vi "meaSureit_SPCM.vi"() -> ()   [LabVIEW 2013]
uses:
  <vilib>/DAQmx/read.llb/DAQmx Read (Analog DBL 1Chan 1Samp).vi
  <vilib>/DAQmx/write.llb/DAQmx Write (Analog DBL 1Chan 1Samp).vi
  <vilib>/DAQmx/read.llb/DAQmx Read (Analog 1D DBL NChan 1Samp).vi
  <vilib>/DAQmx/miscellaneous.llb/DAQmx Fill In Error Info.vi
  <vilib>/Utility/file.llb/Write To Spreadsheet File (DBL).vi
  Instance           2 17Saved   meaSureit .vi
panel:
  in  "Switched":bool=TRUE
  out "Elapsed Time (s)":dbl=22.996299266815186
  in  "Wait time":dbl=60.0 caption="Time Target (s)"
  in  "Auto measurement?":bool
  in  "# sweeps to do":dbl=5.0
  out "Sweeps Completed":dbl
  in  "Sweep":bool
  in  "Auto-pick Sens?":bool
  in  "Auto-pick min. sensitivity":T1(ring)=enum."10nA/V"
  in  "Multiscan Ramp time":dbl=0.5
  in  "Sens Change wait time (ms)":u32=500
  in  "Detect Sens?":bool=TRUE
  in  "Preamp Bias (mv)":i32=-25
  in  "Preamp Bias on?":bool
  in  "Preamp resource":refnum<visa-resource-name>="COM14"
  in  "Preamp Sensitivity":T1(ring)=enum."10nA/V"
  in  "Direction":bool=TRUE
  in  "Cont. Update":bool=TRUE
  out "Error":errorcluster
  in  "Print":bool
  in  "Pause":bool=TRUE caption="Run"
  out "Extension":i32 format="%03.0f"
  in  "Path":path=path "C:/Users/aspitarl/Desktop/a"
  in  "Autosave":bool caption="+"
  in  "Tab Control":T2(tab)
  in  "Parameters":T3={"min"=-10.0, "max"=10.0, "step"=0.03, "speed (steps/s)"=100.0, "Stop at \nthe end"=FALSE} {"step" format="%.5p"; "speed (steps/s)" format="%.2f"; "max" format="%.5p"; "min" format="%.5p"}
  out "end":bool
  in  "Scan Channel 2":u16(ring)=1 items=["Vsd", "Vg", "Time"]
  in  "Scan Channel 3":u16(ring)=1 items=["Vsd", "Vg", "Time"]
  in  "Scan 3":bool caption="+"
  out "value 2":dbl=0.27999999999999997 format="%.5p"
  out "value 3":dbl format="%#.5p"
  in  "delay 3":dbl format="%#.2p"
  in  "delay 2":dbl format="%#.2p"
  in  "Scan":dbl[][](array[numeric])
  out "Value":dbl=0.01000000000002041 format="%#.5p"
  out "graph data":dbl[][](array[numeric]) format="%.2f"
  in  "SaveCFG":bool
  in  "LoadCFG":bool
  in  "update graph":bool=TRUE
  in  "graph bin":dbl=1.0
  out "date":string="Mon, 25 Jul 2016; 13:06"
  out "Data Size":dbl(slide)=228.0 scale=0.0..50000.0 scale format="%.0p"
  in  "Clear":bool
  in  "File Name":string="test"
  in  "Scan Channel":u16(ring)=1 items=["Vsd", "Vg", "Time"]
  in  "Update":bool
  in  "Channels Out":T4(array[cluster])=[{"Channel"=1, "Value"=0.0, "Factor"=1.0, "Name"="Vsd", "min"=-1.0, "max"=1.0, "step"=0.01, "speed"=5.0, "Direction"=TRUE, "Stop at \nthe end"=TRUE}, {"Channel"=2, "Value"=0.01000000000002041, "Factor"=1.0, "Name"="Vg", "min"=-10.0, "max"=10.0, "step"=0.03, "speed"=100.0, "Direction"=TRUE, "Stop at \nthe end"=FALSE}, {"Channel"=0, "Value"=0.0, "Factor"=1.0, "Name"="Time", "min"=0.0, "max"=100000.0, "step"=0.01, "speed"=100.0, "Direction"=FALSE, "Stop at \nthe end"=TRUE}] {"step" format="%.5p"; "speed" format="%.2f"; "max" format="%.5p"; "min" format="%.5p"; "Factor" format="%.2p"; "Value" format="%.5p"}
  out "data":dbl[][](array[numeric]) format="%.2f"
  in  "Y channel":i32(ring) items=["I", "AI2"]
  in  "Save":bool
  out "XY Graph":cluster{dbl[], dbl[]}(graph)
  in  "Quit":bool
  in  "Scan DAQ":bool
  in  "Channels In":T5(array[cluster])=[{"Ring"=1, "Value"=1.691596709266448e-13, "Factor"=1e-09, "Name"="I"}, {"Ring"=2, "Value"=-0.0001533531911967702, "Factor"=1.0, "Name"="AI2"}] {"Factor" format="%.2p"; "Value" format="%.5p"}
  # "speed (steps/sec)"
  # "Direction"
  # "Factor"
  # "Name"
  # "Value"
  # "Factor"
  # "Name"
  # "min"
  # "max"
  # "step"
  # "Value"
  # "Define parameters in the Channels Out Panel"
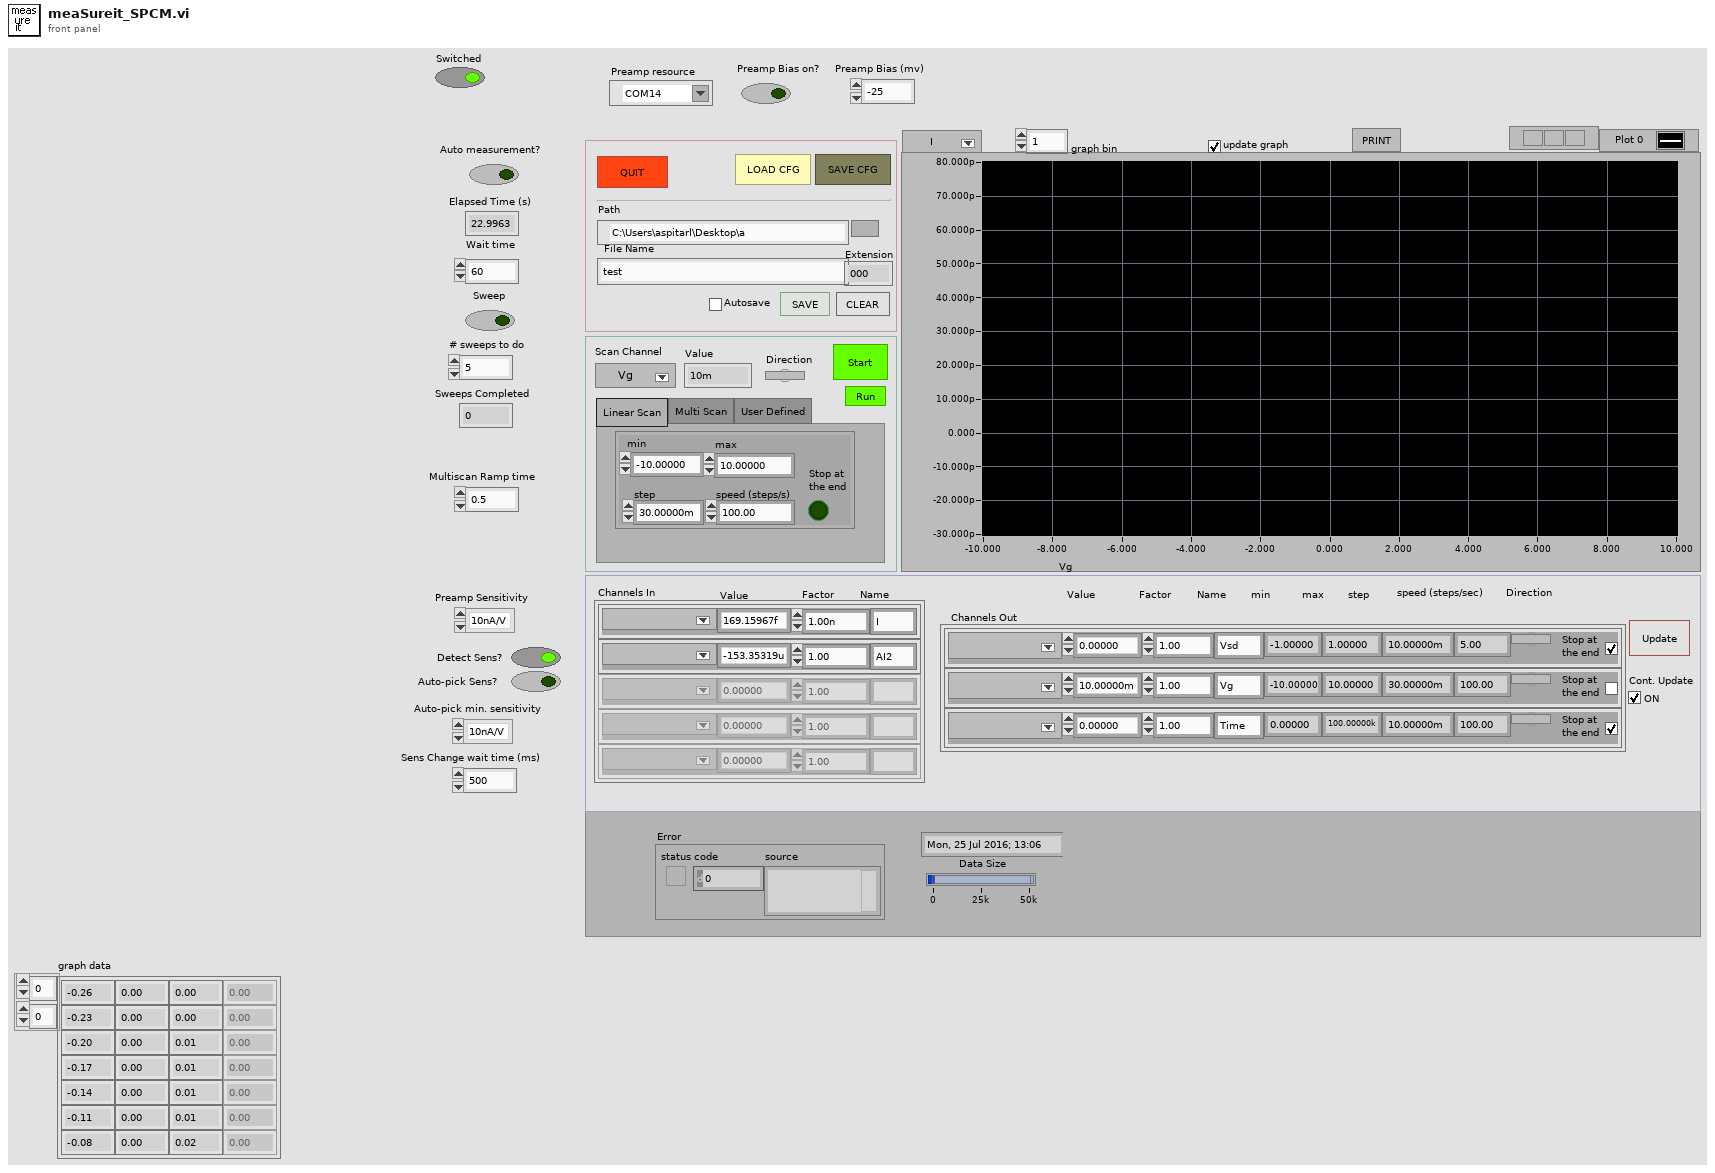
[diagram p1: front panel]
types:
  T1 = enum16{"1pA/V", "2pA/V", "5pA/V", "10pA/V", "20pA/V", "50pA/V", "100pA/V", "200pA/V", "500pA/V", "1nA/V", "2nA/V", "5nA/V", "10nA/V", "20nA/V", "50nA/V", "100nA/V", "200nA/V", "500nA/V", "1uA/V", "2uA/V", "5uA/V", "10uA/V", "20uA/V", "50uA/V", "100uA/V", "200uA/V", "500uA/V", "1mA/V"}
  T2 = enum32{"Linear Scan", "Multi Scan", "User Defined"}
  T3 = cluster{"min":dbl, "max":dbl, "step":dbl, "speed (steps/s)":dbl, "Stop at \nthe end":bool}
  T4 = cluster{"Channel":u16, "Value":dbl, "Factor":dbl, "Name":string, "min":dbl, "max":dbl, "step":dbl, "speed":dbl, "Direction":bool, "Stop at \nthe end":bool}[]
  T5 = cluster{"Ring":u16, "Value":dbl, "Factor":dbl, "Name":string}[]
  T6 = cluster{"Channel":u16, "Value":dbl, "Factor":dbl, "Name":string, "min":dbl, "max":dbl, "step":dbl, "speed":dbl, "direction":bool, "Boolean":bool}[]
  T7 = cluster{"Channel":u16, "Value":dbl, "Factor":dbl, "Name":string}[]
  T8 = cluster{"Channel":u16, "Value":dbl, "Factor":dbl, "Name":string, "min":dbl, "max":dbl, "step":dbl, "speed":dbl, "Direction":bool, "Stop at \nthe end":bool}
  T9 = cluster{"min":dbl, "max":dbl, "step":dbl, "speed (steps/s)":dbl, bool}
  T10 = cluster{void, void, void, void, void, "y":dbl, void, void, void, bool}
  T11 = cluster{void, void, void, void, "y":dbl, void, void, void, void, bool}
  T12 = cluster{void, void, void, void, "y":dbl, void, void, void, void, bool}[]
  T13 = cluster{"Preamp Bias on?":bool, "Preamp Bias (mv)":i32, "Preamp Sensitivity":enum16{"1pA/V", "2pA/V", "5pA/V", "10pA/V", "20pA/V", "50pA/V", "100pA/V", "200pA/V", "500pA/V", "1nA/V", "2nA/V", "5nA/V", "10nA/V", "20nA/V", "50nA/V", "100nA/V", "200nA/V", "500nA/V", "1uA/V", "2uA/V", "5uA/V", "10uA/V", "20uA/V", "50uA/V", "100uA/V", "200uA/V", "500uA/V", "1mA/V"}, "Detect Sens?":bool, "Sens Change wait time (ms)":u32, "Auto-pick min. sensitivity":enum16{"1pA/V", "2pA/V", "5pA/V", "10pA/V", "20pA/V", "50pA/V", "100pA/V", "200pA/V", "500pA/V", "1nA/V", "2nA/V", "5nA/V", "10nA/V", "20nA/V", "50nA/V", "100nA/V", "200nA/V", "500nA/V", "1uA/V", "2uA/V", "5uA/V", "10uA/V", "20uA/V", "50uA/V", "100uA/V", "200uA/V", "500uA/V", "1mA/V"}, "Auto-pick Sens?":bool}
  T14 = cluster{"min":dbl, "max":dbl, "step":dbl, "speed":dbl, "Stop at \nthe end":bool}
  T15 = cluster{"y":dbl, "max":dbl, "step":dbl, "speed (steps/s)":dbl, bool}
  T16 = cluster{"min":dbl, "y":dbl, "step":dbl, "speed (steps/s)":dbl, bool}
  T17 = cluster{"Ring":u16, "Value":dbl, "Factor":dbl, "Name":string}
  T18 = cluster{"Channel":u16, "Value":dbl, "Factor":dbl, "Name":string, "min":dbl, "max":dbl, "step":dbl, "speed":dbl, "Direction":bool, "Stop at the end":bool}[]
  T19 = cluster{"Channel":u16, "Value":dbl, "Factor":dbl, "Name":string, "min":dbl, "max":dbl, "step":dbl, "speed":dbl, "Direction":bool, "Stop at the end":bool}
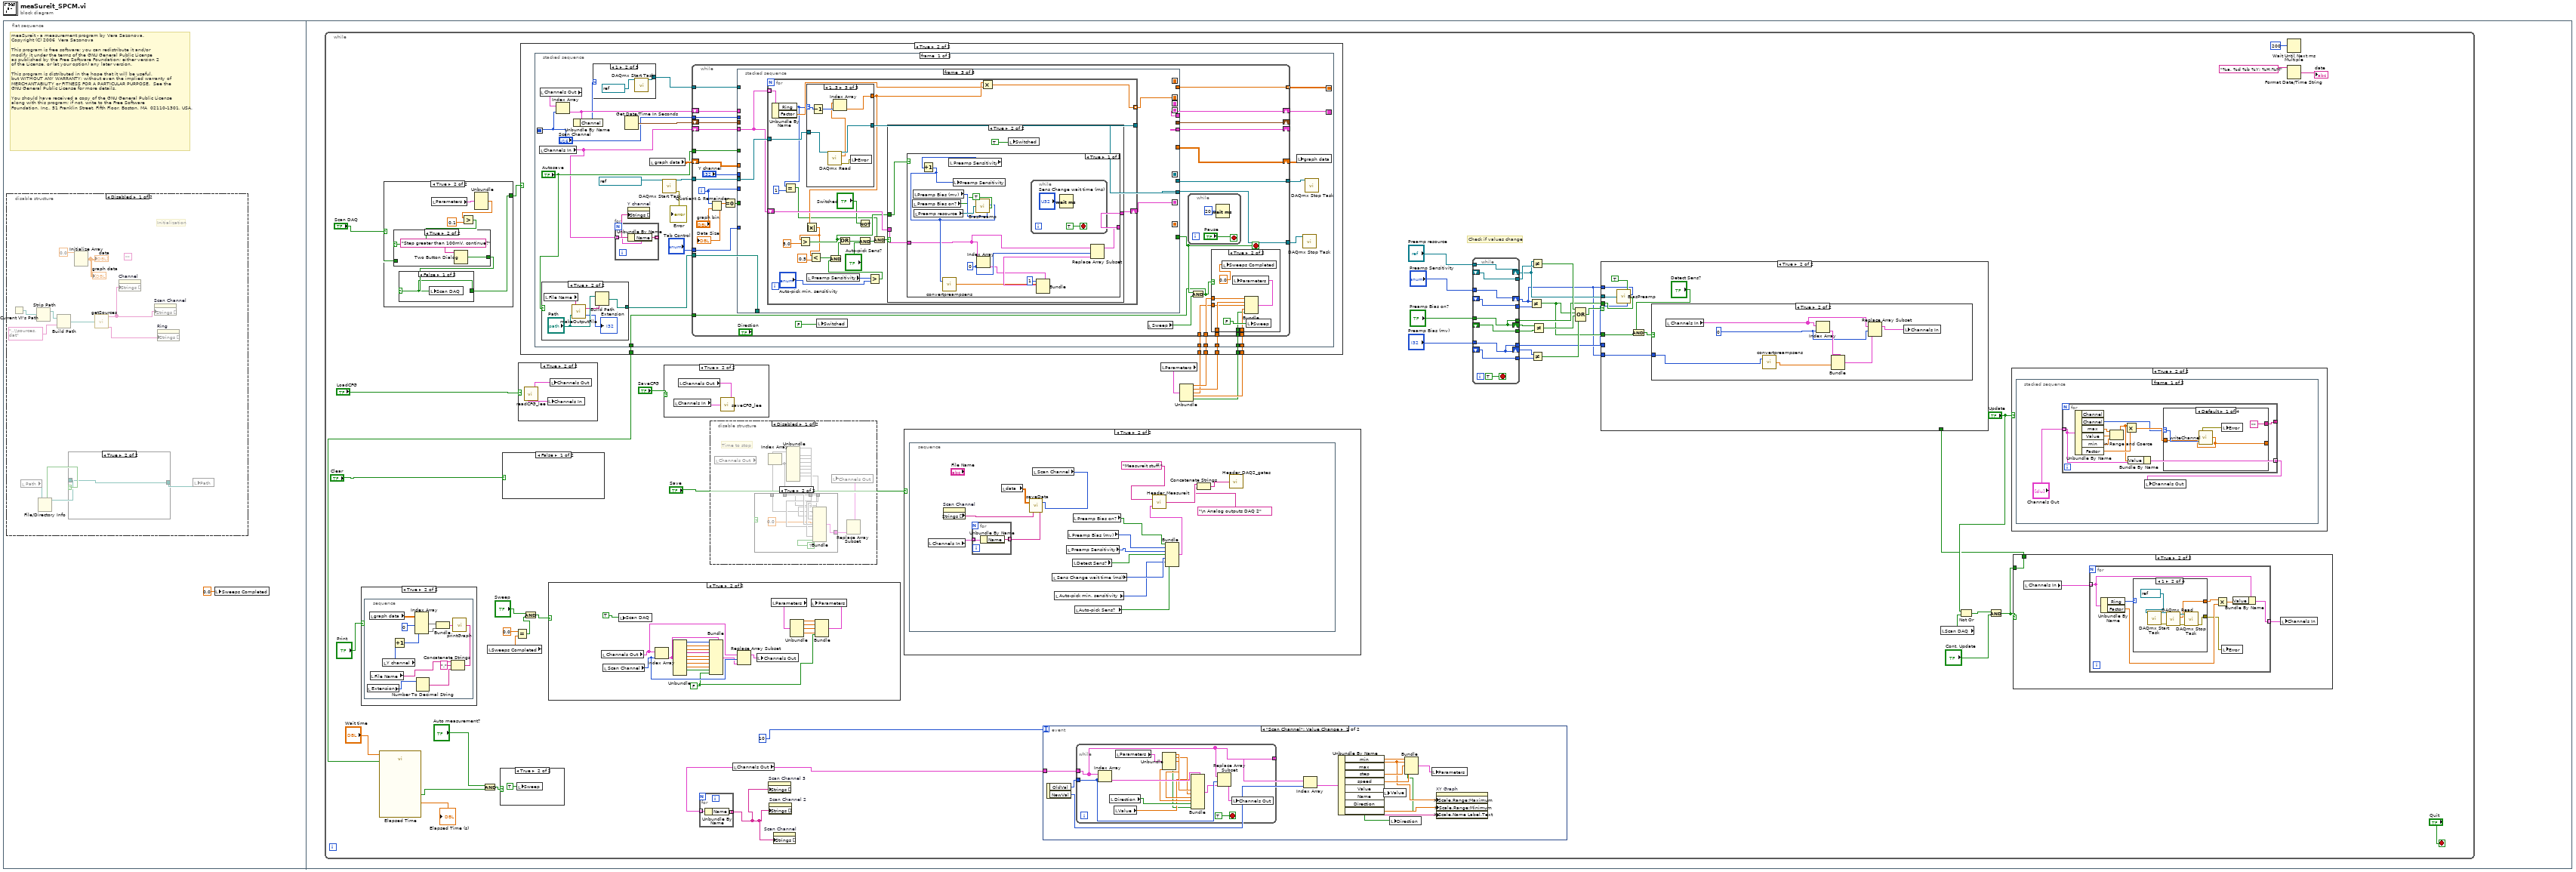
[diagram p0: block diagram]
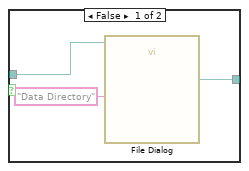
[diagram p2: hidden frame]
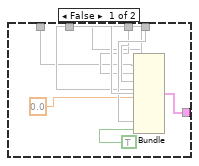
[diagram p5: hidden frame]
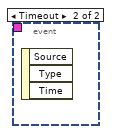
[diagram p13: hidden frame]
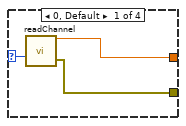
[diagram p15: hidden frame]
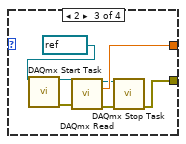
[diagram p16: hidden frame]
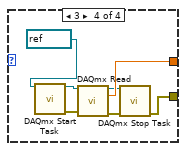
[diagram p17: hidden frame]
diagram:
  n1 = flat-sequence {
    frame #0 {
      # "meaSureit - a measurement program by Vera Sazonova.\nCopyright (C) 2006  Vera Sazonova\n\nThis program is free software; you can redistribute it and/or\nmodify it under the terms of the GNU General Public License\nas published by the Free Software Foundation; either version 2\nof the License, or (at your option) any later version.\n\nThis program is distributed in the hope that it will be useful,\nbut WITHOUT ANY WARRANTY; without even the implied warranty of\nMERCHANTABILITY or FITNESS FOR A PARTICULAR PURPOSE.  See the\nGNU General Public License for more details.\n\nYou should have received a copy of the GNU General Public License\nalong with this program; if not, write to the Free Software\nFoundation, Inc., 51 Franklin Street, Fifth Floor, Boston, MA  02110-1301, USA."
      n2 = disable-structure shown="Disabled" {
        frame Disabled {
          (unwired) ""
          # "Initialization"
          n3 = Current VI's Path() -> (path=w11:path)
          n4 = local read "Path"() -> (w6:path)
          n5 = Strip Path(path=w11) -> (stripped path=w10:path)  [unwired: 1 out]
          n6 = File/Directory Info(path=w6) -> (path out=w4:path, directory=w5:bool)  [unwired: 1 in, 5 out]
          n7 = Build Path(base path=w10, name or relative path="..\\sources.dat") -> (appended path=w2:path)
          n8 = case shown="True" w5 {
            tunnel: w4 -> [w16 w17]
            tunnel: [w15 w17] -> w3
            frame False {
              n9 = call "File Dialog"("start path"=w16, "prompt"="Data Directory") -> ("selected path"=w15:path)  [unwired: 5 in, 8 out]
            }
            frame True {
            }
          }
          n10 = Initialize Array(0.0) -> (→"data" →"graph data":dbl[][])  [unwired: 2 out]
          n11 = call "getSources.vi"("Path"=w2) -> ("Output Sources"=w7:string[], "Input Sources"=w8:string[])  [unwired: 2 out]
          n12 = property on="Channel" class="Ring (strict)"("Strings []"=w7) -> ()  [unwired: 2 in, 2 out]
          n13 = property on="Scan Channel" class="Ring (strict)"("Strings []"=w7) -> ()  [unwired: 2 in, 2 out]
          n14 = property on="Ring" class="Ring (strict)"("Strings []"=w8) -> ()  [unwired: 2 in, 2 out]
          n15 = local write "Path"(w3) -> ()
        }
        frame Enabled {
        }
      }
      n16 = local write "Sweeps Completed"(0.0 ("Number of sweeps")) -> ()
    }
    frame #1 {
      n17 = while {
        stop <- "Quit" stop-if-true
        # "Check if values change"
        n18 = case shown="True" "Print" {
          frame False {
          }
          frame True {
            n19 = stacked-sequence {
              frame #0 {
                n20 = local read "Extension"() -> (w243:i32)
                n21 = local read "graph data"() -> (w246:dbl[][])
                n22 = local read "File Name"() -> (w242:string)
                n23 = local read "Y channel"() -> (w245:i32)
                n24 = Increment(x=w245) -> (x+1=w247:i32)
                n25 = Index Array(array=w246, index (col) #1=0, index (col) #2=w247) -> (element #1=w250:dbl[], element #2=w249:dbl[])  [unwired: 2 in]
                n26 = Number To Decimal String(number=w243) -> (decimal integer string=w240:string)  [unwired: 1 out]
                n27 = Bundle("graph data"=w250, "graph data"=w249) -> (w244:cluster{"graph data":dbl[], "graph data":dbl[]})  [unwired: 1 out]
                n28 = Concatenate Strings(w242, "." ("string"), w240) -> (w239:string)
                n29 = call "printGraph.vi"("File"=w239, "XY Graph 2"=w244) -> ()
              }
            }
          }
        }
        n30 = case shown="True" "Scan DAQ" {
          selector: "Scan DAQ" -> [w136 w139]
          tunnel: [w136 w137] -> w35
          frame False {
          }
          frame True {
            n31 = local read "Parameters"() -> (w143:T3)
            n32 = Unbundle(w143) -> ("step"=w142:dbl)  [unwired: 4 out]
            n33 = Greater?(x=w142, y=0.1) -> (0:w140:bool)
            n34 = case shown="True" w140 {
              tunnel: [w146 w147] -> w138
              tunnel: w139 -> [w146 _]
              frame False {
              }
              frame True {
                n35 = Two Button Dialog(message="Step greater than 100mV, continue?") -> (T button?=w147:bool)  [unwired: 2 in]
              }
            }
            n36 = case shown="False" w138 {
              selector: w138 -> [w144 w145]
              tunnel: [w144 w145] -> w137
              frame False {
                n37 = local write "Scan DAQ"(w144) -> ()
              }
              frame True {
              }
            }
          }
        }
        n38 = local read "Sweeps Completed"() -> (w33:dbl)
        n39 = case shown="False" "Clear" {
          frame False {
          }
          frame True {
            w256 = 0.0
            n40 = local write "Data Size"(w256) -> ()
            n41 = Initialize Array(w256) -> (w255:dbl[][])  [unwired: 2 out]
            n42 = local write "graph data"(w255) -> ()
            n43 = local write "data"(w255) -> ()
          }
        }
        n44 = Equal?(x=0.0, y=w33) -> (x = y?=w31:bool)
        n45 = case shown="True" "LoadCFG" {
          frame False {
          }
          frame True {
            n46 = call "readCFG_lee.vi"() -> ("Channels Out"=w254:T6, "Channels In"=w253:T7)  [unwired: 1 in]
            n47 = local write "Channels In"(w253) -> ()
            n48 = local write "Channels Out"(w254) -> ()
          }
        }
        n49 = And(x="Sweep", y=w31) -> (x .and. y?=w34:bool)
        n50 = case shown="True" w34 {
          frame False {
          }
          frame True {
            w115 = FALSE
            n51 = local read "Channels Out"() -> (w123:T4)
            n52 = local read "Scan Channel"() -> (w125:u16)
            n53 = local write "Scan DAQ"(TRUE) -> ()
            n54 = Index Array(array=w123, index=w125) -> (element=w116:T8)
            n55 = Unbundle(w116) -> ("Channel"=w126:u16, "Value"=w127:dbl, "Factor"=w128:dbl, "Name"=w129:string, "min"=w130:dbl, "max"=w131:dbl, "step"=w132:dbl, "speed"=w133:dbl, "Direction"=w134:bool)  [unwired: 1 out]
            n56 = Bundle(cluster=w116, "Channel"=w126, "Value"=w127, "Factor"=w128, "Name"=w129, "min"=w130, "max"=w131, "step"=w132, "speed"=w133, "Direction"=w134, "Stop at \nthe end"=w115) -> (w124:T8)
            n57 = Replace Array Subset(array=w123, new element=w124, index=w125) -> (w122:T4)
            n58 = local write "Channels Out"(w122) -> ()
            n59 = local read "Parameters"() -> (w121:T3)
            n60 = Unbundle(w121) -> ("min"=w118:dbl, "max"=w119:dbl, "step"=w120:dbl, "speed (steps/s)"=w117:dbl)  [unwired: 1 out]
            n61 = Bundle("min"=w118, "max"=w119, "step"=w120, "speed (steps/s)"=w117, w115) -> (w114:T9)  [unwired: 1 in]
            n62 = local write "Parameters"(w114) -> ()
          }
        }
        n63 = case shown="True" "SaveCFG" {
          frame False {
          }
          frame True {
            n64 = local read "Channels In"() -> (w251:T5)
            n65 = local read "Channels Out"() -> (w252:T4)
            n66 = call "saveCFG_lee.vi"("Channels Out"=w252, "Channels In"=w251) -> ()
          }
        }
        n67 = disable-structure shown="Disabled" {
          frame Disabled {
            # "Time to stop"
            n68 = local read "Channels Out"() -> (w88:T4)
            n69 = Index Array() -> (element=w75)  [unwired: 2 in]
            n70 = Unbundle(w75) -> (w83, w84, w82, w81, w80, w79, w78, w77, w76)  [unwired: 1 out]
            n71 = case shown="True" {
              selector: _ -> [_ _]
              tunnel: w75 -> [w101 w113]
              tunnel: w76 -> [w100 w112]
              tunnel: w77 -> [w99 w111]
              tunnel: w78 -> [w98 w110]
              tunnel: w79 -> [_ w109]
              tunnel: w80 -> [w97 _]
              tunnel: w81 -> [w96 w108]
              tunnel: w82 -> [w95 w107]
              tunnel: w83 -> [w94 w106]
              tunnel: w84 -> [w92 w104]
              tunnel: [w90 w102] -> w85
              frame False {
                n72 = Bundle(cluster=w101, w94, w92, w95, w96, w97, "y"=0.0, w98, w99, w100, TRUE) -> (w90:T10)
              }
              frame True {
                n73 = Bundle(cluster=w113, w106, w104, w107, w108, "y"=0.0, w109, w110, w111, w112, TRUE) -> (w102:T11)
              }
            }
            n74 = Replace Array Subset(new element=w85) -> (array=w87:T12, w89:T12, index=w86:i32)
            n75 = local write "Channels Out"(w89) -> ()
          }
          frame Enabled {
          }
        }
        n76 = local read "Channels Out"() -> (w59:T4)
        n77 = for {
          tunnel: w59 -> [w203] mode=indexing
          tunnel: [w202] -> w58 mode=indexing
          n78 = Unbundle By Name(w203) -> ("Name"=w202:string)
        }
        n79 = property on="Scan Channel 3" class="Ring (strict)"("Strings []"=w58) -> ()  [unwired: 2 in, 2 out]
        n80 = property on="Scan Channel 2" class="Ring (strict)"("Strings []"=w58) -> ()  [unwired: 2 in, 2 out]
        n81 = property on="Scan Channel" class="Ring (strict)"("Strings []"=w58) -> ()  [unwired: 2 in, 2 out]
        n82 = case shown="True" "Save" {
          frame False {
          }
          frame True {
            n83 = stacked-sequence {
              frame #0 {
                n84 = local read "Channels In"() -> (w328:T5)
                n85 = property on="Scan Channel" class="Ring (strict)"() -> ("Strings []"=w330:string[])  [unwired: 2 in, 2 out]
                n86 = for {
                  tunnel: w328 -> [w332] mode=indexing
                  tunnel: [w331] -> w327 mode=indexing
                  n87 = Unbundle By Name(w332) -> ("Name"=w331:string)
                }
                n88 = local read "data"() -> (w329:dbl[][])
                n89 = local read "Scan Channel"() -> (w326:u16)
                n90 = call "saveData.vi"("Names  In"=w327, "Channel"=w326, "Names  Out"=w330, "Data"=w329) -> ()
                n91 = local read "Sens Change wait time (ms)"() -> (w319:u32)
                n92 = local read "Auto-pick min. sensitivity"() -> (w318:T1)
                n93 = local read "Preamp Sensitivity"() -> (w322:T1)
                n94 = local read "Preamp Bias (mv)"() -> (w323:i32)
                n95 = local read "Detect Sens?"() -> (w321:bool)
                n96 = local read "Preamp Bias on?"() -> (w324:bool)
                n97 = local read "Auto-pick Sens?"() -> (w317:bool)
                n98 = Bundle("Preamp Bias on?"=w324, "Preamp Bias (mv)"=w323, "Preamp Sensitivity"=w322, "Detect Sens?"=w321, "Sens Change wait time (ms)"=w319, "Auto-pick min. sensitivity"=w318, "Auto-pick Sens?"=w317) -> (w320:T13)  [unwired: 1 in]
                n99 = call "Header_Measureit.vi"("Cluster"=w320, "String in"="Measureit stuff:") -> ("String out"=w316:string)
                n100 = Concatenate Strings(w316, "\n Analog outputs DAQ 2") -> (w314:string)
                n101 = call "Header_DAQ2_gates.vi"("String in"=w314) -> ()  [unwired: 1 out]
              }
            }
          }
        }
        n102 = event shown="[0] \"Scan Channel\": Value Change" {
          selector: _ -> [_ _]
          dyn-events: _ -> [_ _]
          timeout: 10 -> [_ _]
          tunnel: w59 -> [w178 _]
          event "Scan Channel": Value Change {
            n103 = event-data() -> ("OldVal"=w176:u16, "NewVal"=w177:u16)  [unwired: 1 out]
            n104 = while {
              tunnel: w178 -> [w190]
              tunnel: w176 -> [w192]
              tunnel: [w190] -> w175
              stop <- TRUE stop-if-true
              n105 = Index Array(array=w190, index=w192) -> (element=w200:T8)
              n106 = local read "Direction"() -> (w194:bool)
              n107 = local read "Value"() -> (w193:dbl)
              n108 = local read "Parameters"() -> (w199:T3)
              n109 = Unbundle(w199) -> ("min"=w198:dbl, "max"=w197:dbl, "step"=w196:dbl, "speed (steps/s)"=w195:dbl, "Stop at \nthe end"=w188:bool)
              n110 = Bundle(cluster=w200, "Value"=w193, "min"=w198, "max"=w197, "step"=w196, "speed"=w195, "Direction"=w194, "Stop at \nthe end"=w188) -> (w191:T8)  [unwired: 3 in]
              n111 = Replace Array Subset(array=w190, new element=w191, index=w192) -> (w189:T4)
              n112 = local write "Channels Out"(w189) -> ()
            }
            n113 = Index Array(array=w175, index=w177) -> (element=w187:T8)
            n114 = Unbundle By Name(w187) -> ("min"=w181:dbl, "max"=w182:dbl, "step"=w185:dbl, "speed"=w184:dbl, "Value"=w186:dbl, "Name"=w180:string, "Direction"=w179:bool, "Stop at \nthe end"=w174:bool)
            n115 = local write "Value"(w186) -> ()
            n116 = local write "Direction"(w179) -> ()
            n117 = Bundle("min"=w181, "max"=w182, "step"=w185, "speed"=w184, "Stop at \nthe end"=w174) -> (w183:T14)  [unwired: 1 out]
            n118 = local write "Parameters"(w183) -> ()
            n119 = property on="XY Graph" class="XYGraph (strict)"("X Scale.Range:Maximum"=w182, "X Scale.Range:Minimum"=w181, "X Scale.Name Label.Text"=w180) -> ()  [unwired: 2 in, 2 out]
          }
          event Timeout {
            n120 = event-data() -> ()  [unwired: 4 out]
          }
        }
        n121 = local read "Parameters"() -> (w30:T3)
        n122 = Unbundle(w30) -> ("min"=w29:dbl, "max"=w28:dbl, "step"=w27:dbl, "speed (steps/s)"=w26:dbl, "Stop at \nthe end"=w25:bool)
        n123 = case shown="True" w35 {
          tunnel: w29 -> [_ w339]
          tunnel: w28 -> [_ w338]
          tunnel: w27 -> [_ w337]
          tunnel: w26 -> [_ w336]
          tunnel: w25 -> [_ w335]
          tunnel: [FALSE w334] -> w18
          frame False {
          }
          frame True {
            n124 = stacked-sequence {
              seq-local: [w362 _] -> [_ w759]
              seq-local: [w365 _] -> [_ w756]
              seq-local: ["Scan Channel" _] -> [_ w755]
              tunnel: w339 -> [w345 _]
              tunnel: w338 -> [w344 _]
              tunnel: w337 -> [w343 _]
              tunnel: w336 -> [w342 _]
              tunnel: w335 -> [w341 _]
              tunnel: [w340 _] -> w334
              frame #0 {
                n125 = local read "Channels In"() -> (w348:T5)
                n126 = local read "Channels Out"() -> (w353:T4)
                n127 = case shown="True" "Autosave" {
                  tunnel: [path "" ("appended path") w373] -> w349
                  frame False {
                  }
                  frame True {
                    n128 = local read "File Name"() -> (w372:string)
                    n129 = call "makeOutputFile.vi"("Path"="Path", "Name"=w372) -> ("Extension"=→"Extension":i32, "File Name"=w370:string)
                    n130 = Build Path(base path="Path", name or relative path=w370) -> (appended path=w373:path)
                  }
                }
                n131 = Index Array(array=w353, index="Scan Channel") -> (element=w359:T8)
                n132 = Unbundle By Name(w359) -> ("Channel"=w358:u16)
                n133 = case shown="1" w358 {
                  tunnel: ["" w375 w377 w379 w381] -> w361
                  frame 0, Default {
                  }
                  frame 1 {
                    n134 = call <vilib>:"DAQmx Start Task.vi"("task/channels in"=refnum<k21> "AO0") -> ("task out"=w375:refnum<k21>)  [unwired: 1 in, 13 out]
                  }
                  frame 2 {
                    n135 = call <vilib>:"DAQmx Start Task.vi"("task/channels in"=refnum<k21> "AO1") -> ("task out"=w377:refnum<k21>)  [unwired: 1 in, 13 out]
                  }
                  frame 12 {
                    n136 = call <vilib>:"DAQmx Start Task.vi"("task/channels in"=refnum<k21> "AO2") -> ("task out"=w379:refnum<k21>)  [unwired: 1 in, 13 out]
                  }
                  frame 13 {
                    n137 = call <vilib>:"DAQmx Start Task.vi"("task/channels in"=refnum<k21> "AO3") -> ("task out"=w381:refnum<k21>)  [unwired: 1 in, 13 out]
                  }
                }
                n138 = for {
                  tunnel: w348 -> [w367] mode=indexing
                  tunnel: [w366] -> w347 mode=indexing
                  n139 = Unbundle By Name(w367) -> ("Name"=w366:string)
                }
                n140 = Get Date/Time In Seconds() -> (seconds since 1Jan1904=w356:timestamp)
                n141 = property on="Y channel" class="Ring (strict)"("Strings []"=w347) -> ()  [unwired: 2 in, 2 out]
                n142 = local read "graph data"() -> (w364:dbl[][])
                n143 = call <vilib>:"DAQmx Start Task.vi"("task/channels in"=refnum<k21> "AI0, AI1, AI2") -> ("task out"=w355:refnum<k21>, "error out"=→"Error":errorcluster)  [unwired: 1 in, 12 out]
                n144 = while {
                  shift-right: [w396] -> w365
                  shift-left: w359 -> [w414]
                  shift-right: [w393] -> w363
                  shift-left: w364 -> [w413]
                  tunnel: [w392] -> w362 mode=indexing
                  tunnel: w355 -> [w412]
                  shift-right: [w410] -> _
                  shift-left: w348 -> [w411]
                  tunnel: w361 -> [w405]
                  tunnel: [w404] -> w360
                  tunnel: [w403] -> w354
                  tunnel: "Tab Control" -> [w402]
                  tunnel: w349 -> [w400]
                  shift-right: [w398] -> _
                  shift-left: w356 -> [w399]
                  tunnel: "Scan Channel" -> [w397]
                  tunnel: "Autosave" -> [w394]
                  tunnel: w345 -> [w389]
                  tunnel: w344 -> [w388]
                  tunnel: w343 -> [w387]
                  tunnel: w342 -> [w386]
                  tunnel: w341 -> [w385]
                  tunnel: [w384] -> w340
                  i -> [w401]
                  stop <- w391 stop-if-true
                  n145 = Quotient & Remainder(x=w401, y="graph bin") -> (x-y*floor(x/y)=w408:dbl, floor(x/y)=→"Data Size":dbl)
                  n146 = Equal To 0?(x=w408) -> (x = 0?=w407:bool)
                  n147 = stacked-sequence {
                    seq-local: [_ _ w521 _ _ _ _ _] -> [_ _ _ w599 w631 _ _ _]
                    seq-local: [w428 _ _ _ _ _ _ _] -> [_ w496 _ w600 w632 _ _ _]
                    seq-local: [_ w502 _ _ _ _ _ _] -> [_ _ _ _ _ w650 _ _]
                    seq-local: [_ _ _ _ _ w649 _ _] -> [_ _ _ _ _ _ w706 _]
                    seq-local: [w432 _ _ _ _ _ _ _] -> [_ w497 _ _ _ _ _ _]
                    seq-local: [w429 _ _ _ _ _ _ _] -> [_ _ _ _ _ w647 _ _]
                    seq-local: [_ _ w519 _ _ _ _ _] -> [_ _ _ w597 _ _ _ _]
                    tunnel: w414 -> [w439 w504 _ _ _ w645 _ w740]
                    tunnel: w413 -> [_ _ _ w605 _ _ _ _]
                    tunnel: w412 -> [_ _ w523 _ _ _ _ _]
                    tunnel: w411 -> [_ _ w520 _ _ _ _ _]
                    tunnel: [_ _ _ w604 _ _ _ _] -> w410
                    tunnel: w407 -> [_ _ _ w603 _ _ _ _]
                    tunnel: w405 -> [w437 _ _ _ _ w653 w708 _]
                    tunnel: [_ _ _ _ _ w646 _ _] -> w404
                    tunnel: [_ _ w522 _ _ _ _ _] -> w403
                    tunnel: w399 -> [w435 _ _ _ _ w651 w707 _]
                    tunnel: w402 -> [w434 w503 _ _ _ w654 w709 _]
                    tunnel: w401 -> [w433 _ _ _ _ _ _ _]
                    tunnel: w400 -> [_ _ _ _ w630 _ _ _]
                    tunnel: [_ _ _ _ _ _ _ w744] -> w391
                    tunnel: [_ _ _ _ _ w652 _ _] -> w398
                    tunnel: w397 -> [_ _ _ _ w629 _ _ _]
                    tunnel: [_ _ _ _ _ _ w705 _] -> w396
                    tunnel: "Y channel" -> [_ _ _ w602 _ _ _ _]
                    tunnel: w394 -> [_ _ _ _ w628 _ _ _]
                    tunnel: [_ _ _ w601 _ _ _ _] -> w393
                    tunnel: [_ _ _ w598 _ _ _ _] -> w392
                    frame #0 {
                      # "stop signal after specified number of sweeps"
                      # "Update Values out Indicator"
                      n148 = Unbundle By Name(w439) -> ("Channel"=w438:u16, "Factor"=w431:dbl)
                      n149 = case shown="\"Linear Scan\", Default" w434 {
                        tunnel: [w469 w473 w475] -> w427
                        tunnel: w439 -> [w466 w472 _]
                        tunnel: [w468 w474 w481] -> w430
                        tunnel: [w467 w471 w480] -> w432
                        tunnel: w433 -> [_ _ w476]
                        frame "Linear Scan", Default {
                          n150 = local read "Direction"() -> (w465:bool)
                          n151 = Unbundle By Name(w466) -> ("speed"=w467:dbl)
                          n152 = Bundle By Name(cluster=w466, "Direction"=w465) -> (w464:T8)
                          n153 = call "update_in_scan_Lee.vi"("Parameters"=w464) -> ("Value"=w468:dbl, "end"=w469:bool, "new direction"=w463:bool)
                          n154 = local write "Direction"(w463) -> ()
                        }
                        frame "Multi Scan" {
                          n155 = Unbundle By Name(w472) -> ("speed"=w471:dbl)
                          n156 = call "update_in_scan_Lee.vi"("Parameters"=w472) -> ("Value"=w474:dbl, "end"=w473:bool, "new direction"=w470:bool)
                          n157 = local write "Direction"(w470) -> ()
                        }
                        frame "User Defined" {
                          n158 = Index Array(array="Scan", index (row) #1=w476, index (col) #1=0 ("disabled index (col)"), index (row) #2=w476, index (col) #2=1 ("disabled index (col)")) -> (element #1=w481:dbl, element #2=w480:dbl)
                          n159 = Array Size(array="Scan") -> (size(s)=w478:i32[])
                          n160 = Index Array(array=w478) -> (element=w477:i32)  [unwired: 1 in]
                          n161 = Greater?(x=w477, y=w476) -> (0:w475:bool)
                        }
                      }
                      "end" <- w427
                      n162 = Multiply(x=w431, y=w430) -> (x*y=w436:dbl)
                      n163 = case shown="1, 2, 12, 13" w438 {
                        selector: w438 -> [w486 _ _]
                        tunnel: w437 -> [_ _ w495]
                        tunnel: ["" "" w494] -> w429
                        tunnel: w436 -> [w485 _ w493]
                        tunnel: [w485 w488 w493] -> w428
                        tunnel: w435 -> [_ w489 _]
                        frame Default {
                          n164 = call "writeChannel.vi"("Value"=w485, "Channel"=w486) -> ("error out"=w484:errorcluster)
                          n165 = local write "Error"(w484) -> ()
                        }
                        frame 0 {
                          n166 = Get Date/Time In Seconds() -> (seconds since 1Jan1904=w490:timestamp)
                          n167 = Subtract(x=w490, y=w489) -> (x-y=w488:dbl)
                        }
                        frame 1, 2, 12, 13 {
                          n168 = call-poly <vilib>:"DAQmx Write.vi"("task/channels in"=w495, "data"=w493) -> ("task out"=w494:refnum<k21>, "error out"=w492:errorcluster)  [unwired: 2 in, 10 out]
                          n169 = local write "Error"(w492) -> ()
                        }
                      }
                      "Value" <- w428
                      n170 = local read "Sweep"() -> (w426:bool)
                      n171 = And(x=w427, y=w426) -> (x .and. y?=w425:bool)
                      n172 = case shown="True" w425 {
                        tunnel: w428 -> [_ w440]
                        frame False {
                        }
                        frame True {
                          n173 = local read "Sweeps Completed"() -> (w445:dbl)
                          n174 = Add(x=w445, y=1.0) -> (x+y=w441:dbl)
                          "Sweeps Completed" <- w441
                          n175 = local write "Sweeps Completed"(w441) -> ()
                          n176 = Greater Or Equal?(x=w441, y="# sweeps to do") -> (x >= y?=w442:bool)
                          n177 = case shown="True" w442 {
                            tunnel: w440 -> [_ w447]
                            frame False {
                            }
                            frame True {
                              n178 = Greater?(x=w447, y=0.0) -> (0:w446:bool)
                              n179 = case shown="True" w446 {
                                frame True {
                                n180 = local read "Parameters"() -> (w455:T3)
                                n181 = Unbundle(w455) -> ("max"=w453:dbl, "step"=w454:dbl, "speed (steps/s)"=w452:dbl)  [unwired: 2 out]
                                n182 = Bundle("y"=0.0, "max"=w453, "step"=w454, "speed (steps/s)"=w452, TRUE) -> (w451:T15)  [unwired: 1 in]
                                n183 = local write "Parameters"(w451) -> ()
                                }
                                frame False {
                                n184 = local read "Parameters"() -> (w462:T3)
                                n185 = Unbundle(w462) -> ("min"=w460:dbl, "step"=w461:dbl, "speed (steps/s)"=w459:dbl)  [unwired: 2 out]
                                n186 = Bundle("min"=w460, "y"=0.0, "step"=w461, "speed (steps/s)"=w459, TRUE) -> (w458:T16)  [unwired: 1 in]
                                n187 = local write "Parameters"(w458) -> ()
                                }
                              }
                            }
                          }
                        }
                      }
                    }
                    frame #1 {
                      n188 = case shown="\"Linear Scan\"" w503 {
                        tunnel: w504 -> [w510 w515 w518]
                        tunnel: [w509 w515 w517] -> w502
                        tunnel: w496 -> [w507 _ w516]
                        frame "Linear Scan" {
                          n189 = local read "Direction"() -> (w506:bool)
                          n190 = Unbundle("Parameters") -> ("min"=w512:dbl, "max"=w513:dbl, "step"=w514:dbl, "speed (steps/s)"=w508:dbl, "Stop at \nthe end"=w505:bool)
                          n191 = Bundle(cluster=w510, "Value"=w507, "min"=w512, "max"=w513, "step"=w514, "speed"=w508, "Direction"=w506, "Stop at \nthe end"=w505) -> (w509:T8)  [unwired: 3 out]
                        }
                        frame "User Defined", Default {
                        }
                        frame "Multi Scan" {
                          n192 = Bundle(cluster=w518, "Value"=w516) -> (w517:T8)  [unwired: 9 out]
                        }
                      }
                      n193 = Divide(x=1000, y=w497) -> (x/y=w501:dbl)
                      n194 = Max & Min(x=w501, y=10.0) -> (max(x,y)=w498:dbl)  [unwired: 1 out]
                      n195 = Wait (ms)(milliseconds to wait=w498) -> ()  [unwired: 1 out]
                    }
                    frame #2 {
                      n196 = for {
                        tunnel: w520 -> [w548] mode=indexing
                        tunnel: w523 -> [w546]
                        tunnel: [w545] -> w522
                        tunnel: [w542] -> w521 mode=indexing
                        shift-right: [w544] -> w519
                        shift-left: w520 -> [w543]
                        n197 = Unbundle By Name(w548) -> ("Ring"=w526:u16, "Factor"=w547:dbl)
                        n198 = Equal?(x=w526, y=u16 1) -> (x = y?=w524:bool)
                        n199 = case shown="1..3" w526 {
                          selector: w526 -> [w587 _ w596]
                          tunnel: [w586 0 w595] -> w532
                          tunnel: w546 -> [w584 w588 w593]
                          tunnel: [w584 w588 w592] -> w545
                          frame Default {
                            n200 = call "readChannel.vi"("Channel"=w587) -> ("Value"=w586:dbl, "error out"=w585:errorcluster)
                            n201 = local write "Error"(w585) -> ()
                          }
                          frame 0 {
                          }
                          frame 1..3 {
                            n202 = Decrement(x=w596) -> (x-1=w594:u16)
                            n203 = call-poly <vilib>:"DAQmx Read.vi"("task/channels in"=w593) -> ("task out"=w592:refnum<k21>, "data"=w591:dbl[], "error out"=w590:errorcluster)  [unwired: 1 in, 11 out]
                            n204 = Index Array(array=w591, index=w594) -> (element=w595:dbl)
                            n205 = local write "Error"(w590) -> ()
                          }
                        }
                        n206 = Absolute Value(x=w532) -> (abs(x)=w531:dbl)
                        n207 = Greater?(x=w531, y=5.0) -> (0:w533:bool)
                        n208 = local read "Preamp Sensitivity"() -> (w535:T1)
                        n209 = Less?(x=w531, y=0.5) -> (x < y?=w537:bool)
                        n210 = Not(x="Switched") -> ()  [unwired: 1 out]
                        n211 = Greater?(x=w535, y="Auto-pick min. sensitivity") -> (0:w538:bool)
                        n212 = And(x=w537, y=w538) -> (x .and. y?=w536:bool)
                        n213 = Or(x=w533, y=w536) -> (x .or. y?=w541:bool)
                        n214 = And(x=w541, y="Auto-pick Sens?") -> (x .and. y?=w528:bool)
                        n215 = And(x=w524, y=w528) -> (x .and. y?=w529:bool)
                        n216 = case shown="True" w529 {
                          tunnel: [w549 w553] -> w544
                          tunnel: w543 -> [w549 w552]
                          tunnel: w533 -> [_ w550]
                          frame False {
                          }
                          frame True {
                            n217 = case shown="True" w550 {
                              tunnel: [w555 w572] -> w553
                              tunnel: w552 -> [w554 w571]
                              frame True {
                                w561 = 0 ("index")
                                n218 = local read "Preamp Bias on?"() -> (w563:bool)
                                n219 = local read "Preamp Bias (mv)"() -> (w564:i32)
                                n220 = local read "Preamp resource"() -> (w565:refnum<visa-resource-name>)
                                n221 = local read "Preamp Sensitivity"() -> (w566:T1)
                                n222 = Increment(x=w566) -> (x+1=w557:T1)
                                n223 = call "convertpreampsens.vi"("Preamp Sensitivity"=w557) -> ("Sensitivity"=w559:dbl)  [unwired: 1 in]
                                n224 = local write "Preamp Sensitivity"(w557) -> ()
                                n225 = call "BiasPreamp.vi"("VISA resource name"=w565, "CHANGE SENS?"=TRUE, "Sensitivity"=w557, "Bias on"=w563, "Bias Voltage (mv)"=w564) -> ()
                                n226 = Index Array(array=w554, index=w561) -> (element=w558:T17)
                                n227 = while {
                                stop <- TRUE stop-if-true
                                n228 = Wait (ms)(milliseconds to wait="Sens Change wait time (ms)") -> ()  [unwired: 1 out]
                                }
                                n229 = Bundle(cluster=w558, "Ring"=u16 1, "Factor"=w559) -> (w560:T17)  [unwired: 2 in]
                                n230 = Replace Array Subset(array=w554, new element=w560, index=w561) -> (w555:T5)
                              }
                              frame False {
                                w577 = 0 ("index")
                                n231 = local read "Preamp Bias on?"() -> (w579:bool)
                                n232 = local read "Preamp Bias (mv)"() -> (w580:i32)
                                n233 = local read "Preamp resource"() -> (w581:refnum<visa-resource-name>)
                                n234 = local read "Preamp Sensitivity"() -> (w570:T1)
                                n235 = Decrement(x=w570) -> (x-1=w569:T1)
                                n236 = call "convertpreampsens.vi"("Preamp Sensitivity"=w569) -> ("Sensitivity"=w575:dbl)  [unwired: 1 in]
                                n237 = local write "Preamp Sensitivity"(w569) -> ()
                                n238 = call "BiasPreamp.vi"("VISA resource name"=w581, "CHANGE SENS?"=TRUE, "Sensitivity"=w569, "Bias on"=w579, "Bias Voltage (mv)"=w580) -> ()
                                n239 = Index Array(array=w571, index=w577) -> (element=w574:T17)
                                n240 = while {
                                stop <- TRUE stop-if-true
                                n241 = local read "Sens Change wait time (ms)"() -> (w582:u32)
                                n242 = Wait (ms)(milliseconds to wait=w582) -> ()  [unwired: 1 out]
                                }
                                n243 = Bundle(cluster=w574, "Ring"=u16 1, "Factor"=w575) -> (w576:T17)  [unwired: 2 in]
                                n244 = Replace Array Subset(array=w571, new element=w576, index=w577) -> (w572:T5)
                              }
                            }
                            n245 = local write "Switched"(TRUE) -> ()
                          }
                        }
                        n246 = Multiply(x=w532, y=w547) -> (x*y=w542:dbl)
                      }
                    }
                    frame #3 {
                      n247 = Build Array (concatenate)(w600, w599) -> (w598:dbl[])
                      n248 = case shown="True" w603 {
                        tunnel: w605 -> [w607 w610]
                        tunnel: [w607 w608] -> w601
                        tunnel: w599 -> [_ w614]
                        tunnel: w597 -> [w606 w612]
                        tunnel: [w606 w613] -> w604
                        tunnel: w602 -> [_ w611]
                        tunnel: w598 -> [_ w609]
                        frame False {
                        }
                        frame True {
                          # "Save data in \"data\" array\nand update the graph"
                          n249 = for {
                            tunnel: [w618] -> w613 mode=indexing
                            tunnel: w612 -> [w617] mode=indexing
                            tunnel: w614 -> [w616] mode=indexing
                            n250 = Bundle By Name(cluster=w617, "Value"=w616) -> (w618:T17)
                          }
                          n251 = Build Array (concatenate)(w610, w609) -> (w608:dbl[][])
                          n252 = case shown="True" "update graph" {
                            tunnel: w608 -> [_ w623]
                            tunnel: w612 -> [_ w622]
                            tunnel: w611 -> [_ w619]
                            frame False {
                            }
                            frame True {
                              n253 = local write "Channels In"(w622) -> ()
                              n254 = Increment(x=w619) -> (x+1=w620:i32)
                              n255 = Index Array(array=w623, index (col) #1=0, index (col) #2=w620) -> (element #1=w626:dbl[], element #2=w625:dbl[])  [unwired: 2 in]
                              n256 = Bundle(w626, w625) -> (→"XY Graph":cluster{dbl[], dbl[]})  [unwired: 1 out]
                            }
                          }
                        }
                      }
                    }
                    frame #4 {
                      # "If continuously saving data\nsave it to the file"
                      n257 = local read "Channels Out"() -> (w627:T4)
                      n258 = case shown="True" w628 {
                        tunnel: w632 -> [_ w642]
                        tunnel: w631 -> [_ w641]
                        tunnel: w630 -> [_ w634]
                        tunnel: w627 -> [_ w637]
                        tunnel: w629 -> [_ w635]
                        frame False {
                        }
                        frame True {
                          n259 = for {
                            tunnel: w637 -> [w644] mode=indexing
                            tunnel: [w643] -> w636 mode=indexing
                            n260 = Unbundle By Name(w644) -> ("Value"=w643:dbl)
                          }
                          n261 = Delete From Array(array=w636, index=w635) -> (array with subset deleted=w633:dbl[])  [unwired: 1 in, 1 out]
                          n262 = Build Array (concatenate)(w642, w641, w633) -> (w640:dbl[])
                          n263 = call-poly <vilib>:"Write To Spreadsheet File.vi"("format (%.3f)"="%.15f", "append to file? (new file:F)"=TRUE, "1D data"=w640, "file path (dialog if empty)"=w634) -> ()  [unwired: 2 in, 3 out]
                        }
                      }
                    }
                    frame #5 {
                      # "megascan outer loop 1"
                      n264 = local read "Channels Out"() -> (w648:T4)
                      n265 = case shown="\"Multi Scan\"" w654 {
                        tunnel: w648 -> [_ w668]
                        tunnel: w653 -> [_ w666]
                        tunnel: [w657 w665] -> w652
                        tunnel: w651 -> [w657 w664]
                        tunnel: w650 -> [w656 w663]
                        tunnel: [w656 w662] -> w649
                        tunnel: w647 -> [w655 w660]
                        tunnel: [w655 w659] -> w646
                        tunnel: w645 -> [_ w658]
                        frame "Linear Scan", Default {
                        }
                        frame "Multi Scan" {
                          n266 = local read "end"() -> (w667:bool)
                          n267 = case shown="True" w667 {
                            selector: w667 -> [w670 _]
                            tunnel: w668 -> [_ w690]
                            tunnel: w666 -> [_ w689]
                            tunnel: [w672 w683] -> w665
                            tunnel: w664 -> [w672 _]
                            tunnel: w663 -> [w671 w687]
                            tunnel: [w671 w675] -> w662
                            tunnel: [w670 w684] -> w661
                            tunnel: w660 -> [w669 w677]
                            tunnel: [w669 w676] -> w659
                            tunnel: w658 -> [_ w682]
                            frame False {
                            }
                            frame True {
                              # "Ramp back to inital point channel 2"
                              n268 = flat-sequence {
                                tunnel: [w704] -> w683
                                frame #0 {
                                n269 = Multiply(x="delay 2", y=1000) -> (x*y=w703:dbl)
                                n270 = Wait (ms)(milliseconds to wait=w703) -> ()  [unwired: 1 out]
                                }
                                frame #1 {
                                n271 = Get Date/Time In Seconds() -> (seconds since 1Jan1904=w704:timestamp)
                                }
                              }
                              n272 = Unbundle(w682) -> ("min"=w681:dbl, "max"=w680:dbl)  [unwired: 8 out]
                              n273 = call "update_in_megascan_Lee.vi"("Channels Out"=w690, "Channel"="Scan Channel 2") -> ("Scan Done"=w684:bool, "Array"=w674:T18, "error out"=w685:errorcluster, "current value"=→"value 2":dbl)
                              n274 = local write "Error"(w685) -> ()
                              n275 = local write "Channels Out"(w674) -> ()
                              n276 = call "reset_channel_Lee.vi"("Channel In"=w687, 2:w689) -> ("Channel Out"=w675:T19, "error out"=w686:errorcluster)
                              n277 = call "Generate Saw_1wave.vi"("start"=w680, "finish"=w681) -> ("V out x"=w678:dbl[])  [unwired: 3 in]
                              n278 = local write "Error"(w686) -> ()
                              n279 = for {
                                N: 999 -> [_]
                                tunnel: w678 -> [w697]
                                tunnel: w677 -> [w694]
                                tunnel: [w693] -> w676
                                tunnel: w675 -> [_]
                                tunnel: w674 -> [_]
                                tunnel: "Multiscan Ramp time" -> [w692]
                                i -> [w700]
                                n280 = Multiply(x=1, y=w700) -> (x*y=w698:i32)
                                n281 = Index Array(array=w697, index=w698) -> (element=w696:dbl)
                                n282 = call-poly <vilib>:"DAQmx Write.vi"("task/channels in"=w694, "data"=w696) -> ("task out"=w693:refnum<k21>, "error out"=w695:errorcluster)  [unwired: 2 in, 10 out]
                                n283 = local write "Error"(w695) -> ()
                                n284 = Wait (ms)(milliseconds to wait=w692) -> ()  [unwired: 1 out]
                              }
                            }
                          }
                          n285 = local write "end"(w661) -> ()
                        }
                      }
                    }
                    frame #6 {
                      # "megasweep outer loop 2"
                      n286 = case shown="\"Multi Scan\"" w709 {
                        tunnel: w708 -> [_ w718]
                        tunnel: w707 -> [_ w717]
                        tunnel: w706 -> [w710 w713]
                        tunnel: [w710 w712] -> w705
                        frame "Linear Scan", Default {
                        }
                        frame "Multi Scan" {
                          n287 = local read "Channels Out"() -> (w711:T4)
                          n288 = local read "end"() -> (w715:bool)
                          n289 = And(x=w715, y="Scan 3") -> (x .and. y?=w716:bool)
                          n290 = case shown="True" w716 {
                            tunnel: w711 -> [_ w735]
                            tunnel: w718 -> [_ w731]
                            tunnel: w717 -> [_ _]
                            tunnel: w713 -> [w719 w727]
                            tunnel: [w719 w726] -> w712
                            frame False {
                            }
                            frame True {
                              n291 = call "update_in_megascan_Lee.vi"("Channels Out"=w735, "Channel"="Scan Channel 3") -> ("Scan Done"=w734:bool, "Array"=w723:T18, "current value"=→"value 3":dbl)  [unwired: 1 out]
                              n292 = local read "Scan Channel 2"() -> (w721:u16)
                              n293 = local write "end"(w734) -> ()
                              n294 = Multiply(x="delay 3", y=1000) -> (x*y=w733:dbl)
                              n295 = Index Array(array=w723, index=w721) -> (element=w725:T19)
                              n296 = case shown="0, Default" w721 {
                                tunnel: ["" refnum<k21> "AO0" ("DAQmx Global Channel") refnum<k21> "AO1" ("DAQmx Global Channel")] -> w720
                                frame 0, Default {
                                }
                                frame 1 {
                                }
                                frame 2 {
                                }
                              }
                              n297 = Wait (ms)(milliseconds to wait=w733) -> ()  [unwired: 1 out]
                              n298 = call "reset_channel_Lee.vi"("Channel In"=w725, 2:w720) -> ("Channel Out"=w724:T19)  [unwired: 1 out]
                              n299 = call "reset_channel_Lee.vi"("Channel In"=w727, 2:w731) -> ("Channel Out"=w726:T19)  [unwired: 1 out]
                              n300 = Replace Array Subset(array=w723, new element=w724, index=w721) -> (w722:T18)
                              n301 = local write "Channels Out"(w722) -> ()
                            }
                          }
                        }
                      }
                    }
                    frame #7 {
                      n302 = local read "Tab Control"() -> (w743:T2)
                      n303 = local read "end"() -> (w741:bool)
                      n304 = Unbundle By Name(w740) -> ("Stop at \nthe end"=w739:bool)
                      n305 = local read "Scan DAQ"() -> (w742:bool)
                      n306 = case shown="\"Linear Scan\", Default" w743 {
                        tunnel: [w748 w750] -> w744
                        tunnel: w742 -> [w747 w751]
                        tunnel: w741 -> [w746 w752]
                        tunnel: w739 -> [w745 _]
                        frame "Linear Scan", Default {
                          n307 = call "stop_scan.vi"("end"=w746, "Stop at \nthe end"=w745, "Scan DAQ"=w747) -> ("Boolean"=w748:bool)
                        }
                        frame "Multi Scan" {
                          n308 = call "stop_scan.vi"("end"=w752, "Stop at \nthe end"=TRUE ("Stop at \nthe end"), "Scan DAQ"=w751) -> ("Boolean"=w750:bool)
                        }
                      }
                    }
                  }
                  n309 = local write "Switched"(FALSE) -> ()
                  n310 = local read "Sweep"() -> (w390:bool)
                  n311 = while {
                    stop <- "Pause" stop-if-true
                    n312 = Wait (ms)(milliseconds to wait=u32 20) -> ()  [unwired: 1 out]
                  }
                  n313 = And(x=w391, y=w390) -> (x .and. y?=w384:bool)
                  n314 = case shown="True" w384 {
                    tunnel: w389 -> [_ w420]
                    tunnel: w388 -> [_ w419]
                    tunnel: w387 -> [_ w418]
                    tunnel: w386 -> [_ w417]
                    tunnel: w385 -> [_ w416]
                    frame False {
                    }
                    frame True {
                      n315 = local write "Sweeps Completed"(0.0 ("y")) -> ()
                      n316 = Bundle("min"=w420, "max"=w419, "step"=w418, "speed (steps/s)"=w417, "Stop at \nthe end"=w416) -> (w422:T3)  [unwired: 1 in]
                      n317 = local write "Parameters"(w422) -> ()
                      n318 = local write "Sweep"(FALSE) -> ()
                    }
                  }
                }
                n319 = local write "graph data"(w363) -> ()
                n320 = call <vilib>:"DAQmx Stop Task.vi"("task/channels in"=w354) -> ()  [unwired: 1 in, 14 out]
                n321 = call <vilib>:"DAQmx Stop Task.vi"("task/channels in"=w360) -> ()  [unwired: 1 in, 14 out]
              }
              frame #1 {
                n322 = local read "Autosave"() -> (w758:bool)
                n323 = local write "Scan DAQ"(FALSE) -> ()
                n324 = local read "Channels Out"() -> (w753:T4)
                n325 = case shown="False" w758 {
                  tunnel: w755 -> [w772 _]
                  tunnel: w759 -> [w763 _]
                  tunnel: w753 -> [w762 _]
                  frame False {
                    n326 = Transpose 2D Array(2D array=w763) -> (transposed array=w767:dbl[][])
                    n327 = local read "data"() -> (w771:dbl[][])
                    n328 = Array Size(array=w767) -> (size(s)=w766:i32[])
                    n329 = Index Array(array=w766, index=1) -> (element=w765:i32)
                    n330 = for {
                      tunnel: [w775] -> w761 mode=indexing
                      tunnel: w765 -> [w774]
                      tunnel: w762 -> [w773] mode=indexing
                      n331 = Unbundle By Name(w773) -> ("Value"=w776:dbl)
                      n332 = Initialize Array(w776, w774) -> (w775:dbl[])
                    }
                    n333 = Delete From Array(array=w761, index (row)=w772) -> (array with subset deleted=w760:dbl[][])  [unwired: 2 in, 1 out]
                    n334 = Build Array (concatenate)(w767, w760) -> (w769:dbl[][])
                    n335 = Transpose 2D Array(2D array=w769) -> (transposed array=w768:dbl[][])
                    n336 = Build Array (concatenate)(w771, w768) -> (w770:dbl[][])
                    n337 = local write "data"(w770) -> ()
                  }
                  frame True {
                  }
                }
                n338 = Replace Array Subset(array=w753, new element=w756, index=w755) -> (w754:T4)
                n339 = local write "Channels Out"(w754) -> ()
              }
            }
          }
        }
        n340 = call "Elapsed Time"("Time Target (s)"="Wait time", "Reset"=w18) -> ("Elapsed Time (s)"=→"Elapsed Time (s)":dbl, "Time has Elapsed"=w21:bool)  [unwired: 10 in, 6 out]
        n341 = And(x="Auto measurement?", y=w21) -> (x .and. y?=w20:bool)
        n342 = case shown="True" w20 {
          frame False {
          }
          frame True {
            n343 = local write "Sweep"(TRUE ("Sweep")) -> ()
          }
        }
        n344 = while {
          tunnel: "Preamp resource" -> [w172]
          shift-right: [w172] -> w43
          shift-left: _ -> [w171]
          tunnel: [w171] -> w56
          tunnel: "Preamp Sensitivity" -> [w170]
          shift-right: [w170] -> w39
          shift-left: _ -> [w169]
          tunnel: [w169] -> w54
          tunnel: "Preamp Bias on?" -> [w166]
          shift-right: [w166] -> w51
          shift-left: _ -> [w168]
          tunnel: [w168] -> w52
          tunnel: "Preamp Bias (mv)" -> [w165]
          shift-right: [w165] -> w48
          shift-left: _ -> [w167]
          tunnel: [w167] -> w49
          tunnel: [w166] -> w42
          tunnel: [w165] -> w41
          stop <- TRUE stop-if-true
        }
        n345 = Not Equal?(x=w39, y=w54) -> (x != y?=w40:bool)
        n346 = Not Equal?(x=w43, y=w56) -> (x != y?=w47:bool)
        n347 = Not Equal?(x=w48, y=w49) -> (x != y?=w45:bool)
        n348 = Not Equal?(x=w51, y=w52) -> (x != y?=w46:bool)
        n349 = Compound Arithmetic op=OR(w47, w40, w46, w45) -> (w44:bool)
        n350 = local read "Scan DAQ"() -> (w65:bool)
        n351 = Not Or(1:w65, 2:"Update") -> (0:w66:bool)
        n352 = And(x=w66, y="Cont. Update") -> (x .and. y?=w38:bool)
        n353 = case shown="True" "Update" {
          frame False {
          }
          frame True {
            n354 = stacked-sequence {
              frame #0 {
                n355 = for {
                  tunnel: "Channels Out" -> [w264] mode=indexing
                  tunnel: [w260] -> _
                  tunnel: [w262] -> w257 mode=indexing
                  n356 = Unbundle By Name(w264) -> ("Channel"=w259:u16, "max"=w268:dbl, "Value"=w266:dbl, "min"=w267:dbl, "Factor"=w265:dbl)  [unwired: 1 out]
                  n357 = In Range and Coerce(upper limit=w268, x=w266, lower limit=w267) -> (coerced(x)=w263:dbl)  [unwired: 1 out]
                  n358 = Multiply(x=w263, y=w265) -> (x*y=w261:dbl)
                  n359 = Bundle By Name(cluster=w264, "Value"=w263) -> (w262:T8)
                  n360 = case shown="Default" w259 {
                    selector: w259 -> [w271 _ _ _]
                    tunnel: ["" "" "" ""] -> w260
                    tunnel: w261 -> [w270 w273 w277 w280]
                    tunnel: [w270 w273 w277 w280] -> _
                    frame Default {
                      n361 = call "writeChannel.vi"("Value"=w270, "Channel"=w271) -> ("error out"=w269:errorcluster)
                      n362 = local write "Error"(w269) -> ()
                    }
                    frame 0 {
                    }
                    frame 1 {
                      n363 = call-poly <vilib>:"DAQmx Write.vi"("task/channels in"=refnum<k21> "AO0", "data"=w277) -> ()  [unwired: 2 in, 12 out]
                    }
                    frame 2 {
                      n364 = call-poly <vilib>:"DAQmx Write.vi"("task/channels in"=refnum<k21> "AO1", "data"=w280) -> ()  [unwired: 2 in, 12 out]
                    }
                  }
                }
                n365 = local write "Channels Out"(w257) -> ()
              }
              frame #1 {
                n366 = for {
                  tunnel: "Channels In" -> [w287] mode=indexing
                  tunnel: [w285] -> w282 mode=indexing
                  n367 = Unbundle By Name(w287) -> ("Ring"=w289:u16, "Factor"=w288:dbl)
                  n368 = case shown="1" w289 {
                    selector: w289 -> [w292 _ _ _]
                    tunnel: [w291 w293 w306 w308] -> w283
                    tunnel: [w290 w294 w300 w309] -> w284
                    frame 0, Default {
                      n369 = call "readChannel.vi"("Channel"=w292) -> ("Value"=w291:dbl, "error out"=w290:errorcluster)
                    }
                    frame 1 {
                      n370 = call <vilib>:"DAQmx Start Task.vi"("task/channels in"=refnum<k21> "AI0") -> ("task out"=w298:refnum<k21>, "error out"=w296:errorcluster)  [unwired: 1 in, 12 out]
                      n371 = call-poly <vilib>:"DAQmx Read.vi"("task/channels in"=w298, "error in"=w296) -> ("task out"=w297:refnum<k21>, "data"=w293:dbl, "error out"=w295:errorcluster)  [unwired: 11 out]
                      n372 = call <vilib>:"DAQmx Stop Task.vi"("task/channels in"=w297, "error in"=w295) -> ("error out"=w294:errorcluster)  [unwired: 13 out]
                    }
                    frame 2 {
                      n373 = call <vilib>:"DAQmx Start Task.vi"("task/channels in"=refnum<k21> "AI1") -> ("task out"=w304:refnum<k21>, "error out"=w302:errorcluster)  [unwired: 1 in, 12 out]
                      n374 = call-poly <vilib>:"DAQmx Read.vi"("task/channels in"=w304, "error in"=w302) -> ("task out"=w303:refnum<k21>, "data"=w306:dbl, "error out"=w301:errorcluster)  [unwired: 11 out]
                      n375 = call <vilib>:"DAQmx Stop Task.vi"("task/channels in"=w303, "error in"=w301) -> ("error out"=w300:errorcluster)  [unwired: 13 out]
                    }
                    frame 3 {
                      n376 = call <vilib>:"DAQmx Start Task.vi"("task/channels in"=refnum<k21> "AI2") -> ("task out"=w312:refnum<k21>, "error out"=w311:errorcluster)  [unwired: 1 in, 12 out]
                      n377 = call-poly <vilib>:"DAQmx Read.vi"("task/channels in"=w312, "error in"=w311) -> ("task out"=w307:refnum<k21>, "data"=w308:dbl, "error out"=w310:errorcluster)  [unwired: 11 out]
                      n378 = call <vilib>:"DAQmx Stop Task.vi"("task/channels in"=w307, "error in"=w310) -> ("error out"=w309:errorcluster)  [unwired: 13 out]
                    }
                  }
                  n379 = Multiply(x=w283, y=w288) -> (x*y=w286:dbl)
                  n380 = local write "Error"(w284) -> ()
                  n381 = Bundle By Name(cluster=w287, "Value"=w286) -> (w285:T17)
                }
                n382 = local write "Channels In"(w282) -> ()
              }
            }
          }
        }
        n383 = case shown="True" w38 {
          tunnel: w38 -> [w204 w205]
          tunnel: [w204 w205] -> w37
          frame False {
          }
          frame True {
            n384 = local read "Channels In"() -> (w207:T5)
            n385 = for {
              tunnel: w207 -> [w212] mode=indexing
              tunnel: [w210] -> w206 mode=indexing
              n386 = Unbundle By Name(w212) -> ("Ring"=w214:u16, "Factor"=w213:dbl)
              n387 = case shown="1" w214 {
                selector: w214 -> [w217 _ _ _]
                tunnel: [w216 w218 w231 w233] -> w208
                tunnel: [w215 w219 w225 w234] -> w209
                frame 0, Default {
                  n388 = call "readChannel.vi"("Channel"=w217) -> ("Value"=w216:dbl, "error out"=w215:errorcluster)
                }
                frame 1 {
                  n389 = call <vilib>:"DAQmx Start Task.vi"("task/channels in"=refnum<k21> "AI0") -> ("task out"=w223:refnum<k21>, "error out"=w221:errorcluster)  [unwired: 1 in, 12 out]
                  n390 = call-poly <vilib>:"DAQmx Read.vi"("task/channels in"=w223, "error in"=w221) -> ("task out"=w222:refnum<k21>, "data"=w218:dbl, "error out"=w220:errorcluster)  [unwired: 11 out]
                  n391 = call <vilib>:"DAQmx Stop Task.vi"("task/channels in"=w222, "error in"=w220) -> ("error out"=w219:errorcluster)  [unwired: 13 out]
                }
                frame 2 {
                  n392 = call <vilib>:"DAQmx Start Task.vi"("task/channels in"=refnum<k21> "AI1") -> ("task out"=w229:refnum<k21>, "error out"=w227:errorcluster)  [unwired: 1 in, 12 out]
                  n393 = call-poly <vilib>:"DAQmx Read.vi"("task/channels in"=w229, "error in"=w227) -> ("task out"=w228:refnum<k21>, "data"=w231:dbl, "error out"=w226:errorcluster)  [unwired: 11 out]
                  n394 = call <vilib>:"DAQmx Stop Task.vi"("task/channels in"=w228, "error in"=w226) -> ("error out"=w225:errorcluster)  [unwired: 13 out]
                }
                frame 3 {
                  n395 = call <vilib>:"DAQmx Start Task.vi"("task/channels in"=refnum<k21> "AI2") -> ("task out"=w237:refnum<k21>, "error out"=w236:errorcluster)  [unwired: 1 in, 12 out]
                  n396 = call-poly <vilib>:"DAQmx Read.vi"("task/channels in"=w237, "error in"=w236) -> ("task out"=w232:refnum<k21>, "data"=w233:dbl, "error out"=w235:errorcluster)  [unwired: 11 out]
                  n397 = call <vilib>:"DAQmx Stop Task.vi"("task/channels in"=w232, "error in"=w235) -> ("error out"=w234:errorcluster)  [unwired: 13 out]
                }
              }
              n398 = Multiply(x=w208, y=w213) -> (x*y=w211:dbl)
              n399 = local write "Error"(w209) -> ()
              n400 = Bundle By Name(cluster=w212, "Value"=w211) -> (w210:T17)
            }
            n401 = local write "Channels In"(w206) -> ()
          }
        }
        n402 = case shown="True" w44 {
          tunnel: w43 -> [_ w156]
          tunnel: w39 -> [_ w155]
          tunnel: w42 -> [_ w154]
          tunnel: w41 -> [_ w153]
          tunnel: w40 -> [_ w151]
          tunnel: w39 -> [_ w149]
          tunnel: w37 -> [_ _]
          frame False {
          }
          frame True {
            n403 = call "BiasPreamp.vi"("VISA resource name"=w156, "CHANGE SENS?"=TRUE, "Sensitivity"=w155, "Bias on"=w154, "Bias Voltage (mv)"=w153) -> ()
            n404 = And(x="Detect Sens?", y=w151) -> (x .and. y?=w150:bool)
            n405 = case shown="True" w150 {
              tunnel: w149 -> [_ w163]
              frame False {
              }
              frame True {
                w161 = 0 ("index")
                n406 = local read "Channels In"() -> (w160:T5)
                n407 = call "convertpreampsens.vi"("Preamp Sensitivity"=w163) -> ("Sensitivity"=w162:dbl)  [unwired: 1 in]
                n408 = Index Array(array=w160, index=w161) -> (element=w164:T17)
                n409 = Bundle(cluster=w164, "Factor"=w162) -> (w159:T17)  [unwired: 3 in]
                n410 = Replace Array Subset(array=w160, new element=w159, index=w161) -> (w158:T5)
                n411 = local write "Channels In"(w158) -> ()
              }
            }
          }
        }
        n412 = Wait Until Next ms Multiple(millisecond multiple=200) -> ()  [unwired: 1 out]
        n413 = Format Date/Time String(time format string (%c)="%a, %d %b %Y; %H:%M") -> (date/time string=→"date":string)  [unwired: 2 out]
      }
    }
  }
